vi "S4PToExcel.vi"(0 "Data Basic Path":path=path "D:/", 1 "Diff S-parameters Data 2":dbl[][][](array[numeric]), 2 "Selected tem":string[](array[string])=["SDD21", "SDD11", "SDD22", "SCC11"], 3 "Pair  Name":string[](array[string]), 4 "Frequency(Hz)":dbl[](array[numeric]), 5 "error in (no error)":errorcluster caption="错误输入（无错误）", 7 "Sample Name":string) -> ()   [LabVIEW 2011]
uses:
  <vilib>/Utility/NIReport.llb/NI_report.lvclass
  <vilib>/addons/_office/excel.llb/Excel Easy Table (str).vi
  <vilib>/Utility/NIReport.llb/Excel/NI_Excel.lvclass
  <vilib>/addons/_office/NI_ReportGenerationToolkit.lvlib
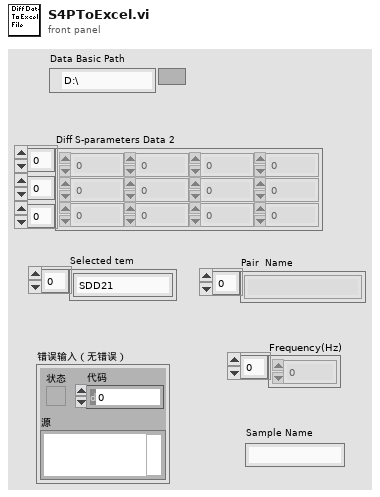
[diagram p1: front panel]
types:
  T1 = enum16{"Standard Report", "HTML", "Word", "Excel"}
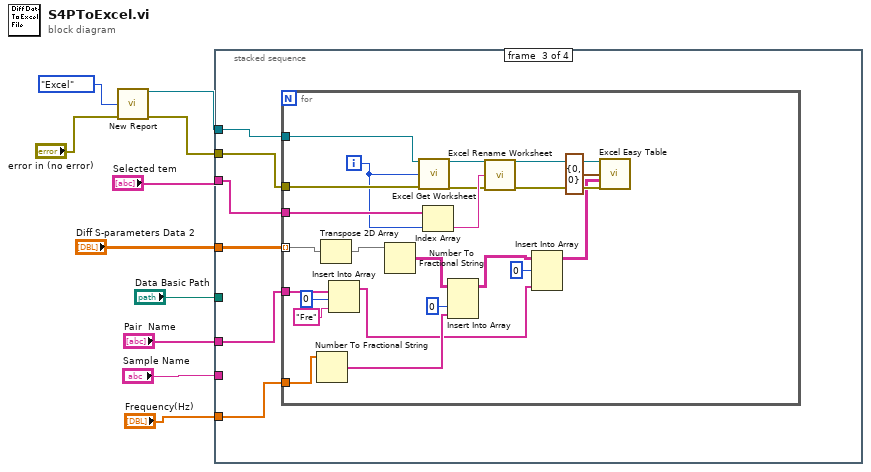
[diagram p0: block diagram]
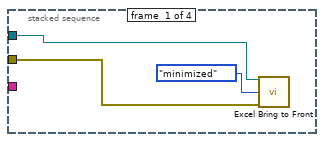
[diagram p2: hidden frame]
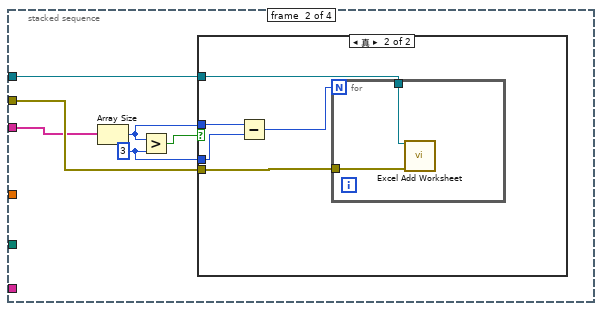
[diagram p3: hidden frame]
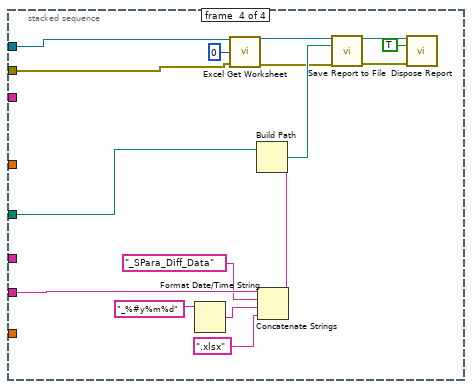
[diagram p5: hidden frame]
diagram:
  n1 = call <vilib>:"New Report.vi"("report type"=T1."Excel", "error in (no error)"="error in (no error)") -> ("report out"=w8:refnum<class "NI_report.lvclass">, "error out"=w7:errorcluster)  [unwired: 12 in]
  n2 = stacked-sequence {
    tunnel: "Selected tem" -> [_ w17 w32 _]
    tunnel: w8 -> [w12 w19 w31 w64]
    tunnel: w7 -> [w11 w18 w30 w63]
    tunnel: "Diff S-parameters Data 2" -> [_ _ w29 _]
    tunnel: "Data Basic Path" -> [_ _ _ w62]
    tunnel: "Pair  Name" -> [_ _ w28 _]
    tunnel: "Frequency(Hz)" -> [_ _ w27 _]
    tunnel: "Sample Name" -> [_ _ _ w61]
    frame #0 {
      n3 = call <vilib>:"Excel Bring to Front.vi"("report in"=w12, "window state (maximized)"=enum16{"maximized", "minimized", "normal"}."minimized", "error in (no error)"=w11) -> ()  [unwired: 11 in, 2 out]
    }
    frame #1 {
      w14 = 3 ("y")
      n4 = Array Size(array=w17) -> (size(s)=w15:i32)
      n5 = Greater?(x=w15, y=w14) -> (0:w16:bool)
      n6 = case shown="真" w16 {
        tunnel: w19 -> [_ w24]
        tunnel: w18 -> [_ w23]
        tunnel: w15 -> [_ w22]
        tunnel: w14 -> [_ w21]
        frame False {
        }
        frame True {
          n7 = Subtract(x=w22, y=w21) -> (x-y=w20:i32)
          n8 = for {
            N: w20 -> [_]
            tunnel: w24 -> [w26]
            tunnel: w23 -> [w25]
            n9 = call <vilib>:"Excel Add Worksheet.vi"("report in"=w26, "error in (no error)"=w25) -> ()  [unwired: 12 in, 2 out]
          }
        }
      }
    }
    frame #2 {
      n10 = for {
        tunnel: w32 -> [w52]
        tunnel: w31 -> [w55]
        tunnel: w30 -> [w54]
        tunnel: w29 -> [w53] mode=indexing
        tunnel: w28 -> [w41]
        tunnel: w27 -> [w38]
        i -> [w51]
        n11 = Number To Fractional String(number=w38) -> (F-format string=w36:string[])  [unwired: 3 in]
        n12 = Transpose 2D Array(2D array=w53) -> (transposed array=w44:dbl[][])
        n13 = Insert Into Array(array=w41, index=0 ("索引"), new element="Fre" ("新元素/子数组")) -> (w33:string[])
        n14 = Number To Fractional String(number=w44) -> (F-format string=w37:string[][])  [unwired: 3 in]
        n15 = call <vilib>:"Excel Get Worksheet.vi"("report in"=w55, "worksheet index (0)"=w51, "error in (no error)"=w54) -> ("report out"=w50:refnum<class "NI_report.lvclass">, "error out"=w48:errorcluster)  [unwired: 11 in]
        n16 = Index Array(array=w52, index=w51) -> (element=w49:string)
        n17 = Insert Into Array(array=w37, index (col)=0 ("禁用的索引 (列)"), new element=w36) -> (w34:string[][])  [unwired: 1 in]
        n18 = call <vilib>:"Excel Rename Worksheet.vi"("report in"=w50, "worksheet name (\"\")"=w49, "error in (no error)"=w48) -> ("report out"=w46:refnum<class "NI_report.lvclass">, "error out"=w47:errorcluster)  [unwired: 11 in]
        n19 = Insert Into Array(array=w34, index (row)=0 ("索引 (行)"), new element=w33) -> (w42:string[][])  [unwired: 1 in]
        n20 = call-poly <vilib>:"Excel Easy Table.vi"("report in"=w46, "start (0, 0)"=cluster{"row":i32, "column":i32} {"row"=0, "column"=0}, "text data"=w42, "error in (no error)"=w47) -> ()  [unwired: 7 in, 5 out]
      }
    }
    frame #3 {
      n21 = Format Date/Time String(time format string (%c)="_%#y%m%d") -> (date/time string=w57:string)  [unwired: 2 in]
      n22 = call <vilib>:"Excel Get Worksheet.vi"("report in"=w64, "worksheet index (0)"=0, "error in (no error)"=w63) -> ("report out"=w65:refnum<class "NI_report.lvclass">, "error out"=w66:errorcluster)  [unwired: 11 in]
      n23 = Concatenate Strings(w61, "_SPara_Diff_Data" ("字符串"), w57, ".xlsx" ("字符串")) -> (w59:string)
      n24 = Build Path(base path=w62, name or relative path=w59) -> (appended path=w67:path)
      n25 = call-dynamic "Save Report to File.vi"("report in"=w65, "report file path"=w67, "error in (no error)"=w66) -> ("report out"=w69:refnum<class "NI_report.lvclass">, "error out"=w70:errorcluster)  [unwired: 11 in]
      n26 = call-dynamic "Dispose Report.vi"("report in"=w69, "wait until printing completed? (T)"=TRUE, "error in (no error)"=w70) -> ()  [unwired: 12 in, 1 out]
    }
  }
